vi "To Variant.vi"(8 "error in":errorcluster, 11 "Assert in":refnum<class "Assertion.lvclass">) -> (0 "error out":errorcluster, 3 "Variant":variant)   [LabVIEW 2020, in "Assertion.lvclass"]
uses:
  <vilib>/gpm_packages/@cs/data-type-serializer/source/Assertion/Assertion.lvclass
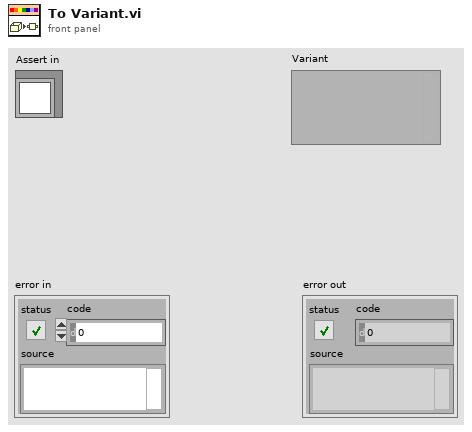
[diagram p1: front panel]
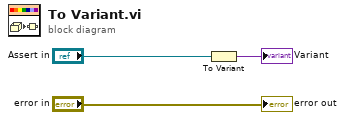
[diagram p0: block diagram]
diagram:
  n1 = To Variant(anything="Assert in") -> (Variant=→"Variant":variant)
  "error out" <- "error in"
